vi "Active Logical Channel.vi"(8 "error in (no error)":errorcluster, 10 "Logical channel State":u16(ring) items=["OFF", "ON"], 11 "VISA resource name":refnum<visa-resource-name>) -> (0 "error out":errorcluster, 3 "VISA resource name out":refnum<visa-resource-name>)   [LabVIEW 2017, in "Sefram DAS220.lvlib"]
doc: "Enable the group of logical channels."
uses:
  <instrlib>/Sefram DAS220/Sefram DAS220.lvlib
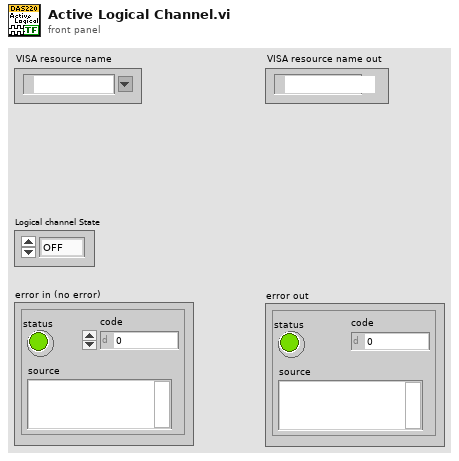
[diagram p1: front panel]
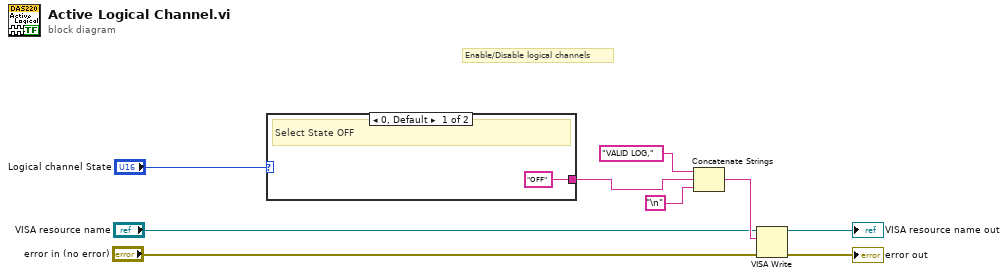
[diagram p0: block diagram]
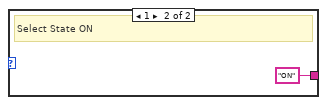
[diagram p2: hidden frame]
diagram:
  # "Enable/Disable logical channels"
  n1 = case shown="0, Default" "Logical channel State" {
    tunnel: ["OFF" "ON"] -> w4
    frame 0, Default {
      # "Select State OFF"
    }
    frame 1 {
      # "Select State ON"
    }
  }
  n2 = Concatenate Strings("VALID LOG," ("write buffer"), w4, "\n") -> (w8:string)
  n3 = VISA Write(VISA resource name="VISA resource name", write buffer=w8, error in (no error)="error in (no error)") -> (VISA resource name out=→"VISA resource name out":refnum<visa-resource-name>, error out=→"error out":errorcluster)  [unwired: 1 out]
